vi "Coerce Temp Setpoint within Limits--SubVI.vi"(8 "error in (no error)":errorcluster, 10 "Temp Setpoint Data":T1, 11 "Watlow F4T in":refnum<class "Watlow F4T.lvclass">) -> (0 "error out":errorcluster, 2 "Temp Setpoint Out":dbl, 3 "Watlow F4T out":refnum<class "Watlow F4T.lvclass">)   [LabVIEW 2024, in "Watlow F4T.lvclass"]
uses:
  Watlow F4T.lvclass
  Process Controller/Controls/Temp Data--Cluster.ctl
  Process Controller/Controls/Temperature Units--Enum.ctl
  Watlow F4T.lvclass/Watlow F4T.ctl
  <vilib>/Utility/error.llb/Error Cluster From Error Code.vi
  <vilib>/ErrorRing/Error Ring.xnode
  Process Controller/_Thermal Process Controller.lvclass
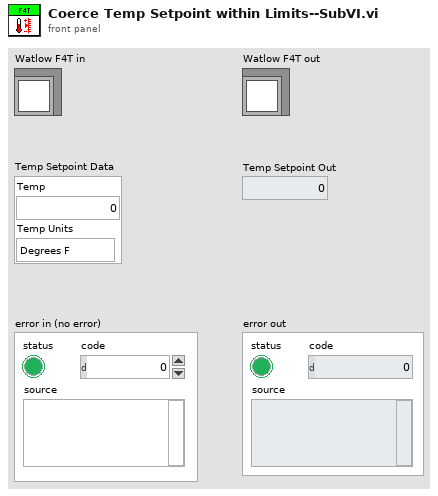
[diagram p1: front panel]
types:
  T1 = typedef "_Thermal Process Controller.lvclass/Temp Data--Cluster.ctl" = cluster{"Temp":dbl, "Temp Units":T2}
  T2 = typedef "_Thermal Process Controller.lvclass/Temperature Units--Enum.ctl" = enum16{"Degrees F", "Degrees C", "Degrees K"}
  T3 = typedef "_Thermal Process Controller.lvclass/Limits--Cluster.ctl" = cluster{"Upper Limit":dbl, "Lower Limit":dbl}
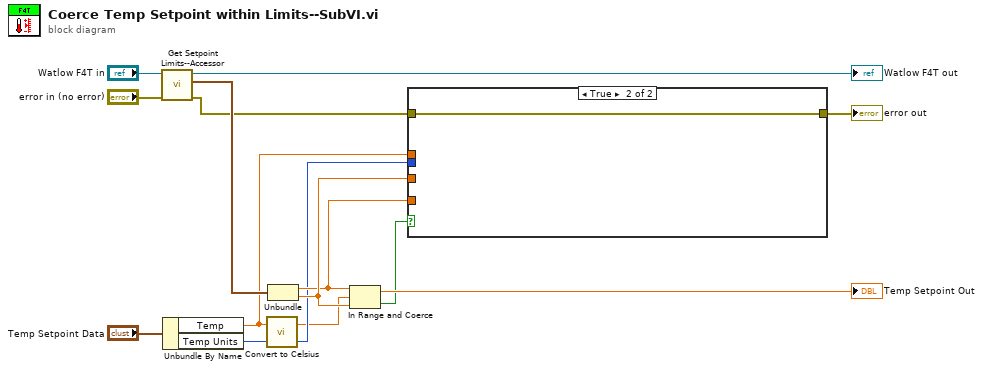
[diagram p0: block diagram]
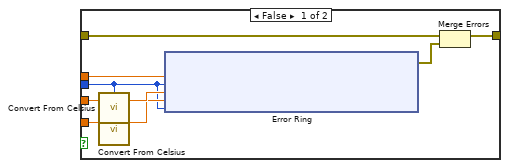
[diagram p2: hidden frame]
diagram:
  n1 = call "Get Setpoint Limits--Accessor.vi"("error in (no error)"="error in (no error)", "Watlow F4T in"="Watlow F4T in") -> ("error out"=w3:errorcluster, "Limits"=w7:T3, "Watlow F4T out"=→"Watlow F4T out":refnum<class "Watlow F4T.lvclass">)  [unwired: 7 in]
  n2 = Unbundle By Name("Temp Setpoint Data") -> ("Temp"=w1:dbl, "Temp Units"=w5:T2)
  n3 = call "Convert to Celsius.vi"("Temp In"=w1, "Temp Units"=w5) -> ("Temp Out"=w4:dbl)  [unwired: 3 in]
  n4 = Unbundle(w7) -> ("Upper Limit"=w11:dbl, "Lower Limit"=w12:dbl)
  n5 = In Range and Coerce(upper limit=w11, x=w4, lower limit=w12) -> (coerced(x)=→"Temp Setpoint Out":dbl, In Range?=w10:bool)
  n6 = case shown="True" w10 {
    tunnel: [w22 w35] -> w14
    tunnel: w11 -> [w19 _]
    tunnel: w12 -> [w18 _]
    tunnel: w5 -> [w16 _]
    tunnel: w1 -> [w17 _]
    tunnel: w3 -> [w15 w35]
    frame False {
      n7 = call "Convert From Celsius.vi"("Temp In"=w18, "Temp Units"=w16) -> ("Temp Out"=w21:dbl)  [unwired: 3 in]
      n8 = call "Convert From Celsius.vi"("Temp In"=w19, "Temp Units"=w16) -> ("Temp Out"=w20:dbl)  [unwired: 3 in]
      n9 = xnode "Error Ring"("parameter 0"=w17, "parameter 1"=w16, "parameter 2"=w21, "parameter 3"=w20, "parameter 4"=w16) -> ("error out"=w23:errorcluster)
      n10 = Merge Errors(w15, w23) -> (w22:errorcluster)
    }
    frame True {
    }
  }
  "error out" <- w14
